vi "Main.vi"() -> ()   [LabVIEW 2009]
uses:
  <vilib>/Instr/_visa.llb/VISA Configure Serial Port (Instr).vi
panel:
  out "x-y":u32
  out "String":string
  in  "偵測數值":bool
  out "Cluster":T1={"試驗速度"=10, "加速時間"=10, "試驗次數"=5000, "輪胎直徑"=1000, "異常煞車時間"=50}
  in  "stop":bool
  in  "偵測開啟":bool
  in  "控制開啟":bool
  in  "Y10~Y17":bool[](array[boolean])=[FALSE, FALSE, FALSE, FALSE, FALSE, FALSE, FALSE, FALSE]
  in  "Y0~Y7":bool[](array[boolean])=[FALSE, FALSE, FALSE, FALSE, FALSE, FALSE, FALSE, FALSE]
  out "X10~X17":bool[](array[boolean])
  out "X0~X7":bool[](array[boolean])
  in  "COM Port":refnum<visa-resource-name>="COM6"
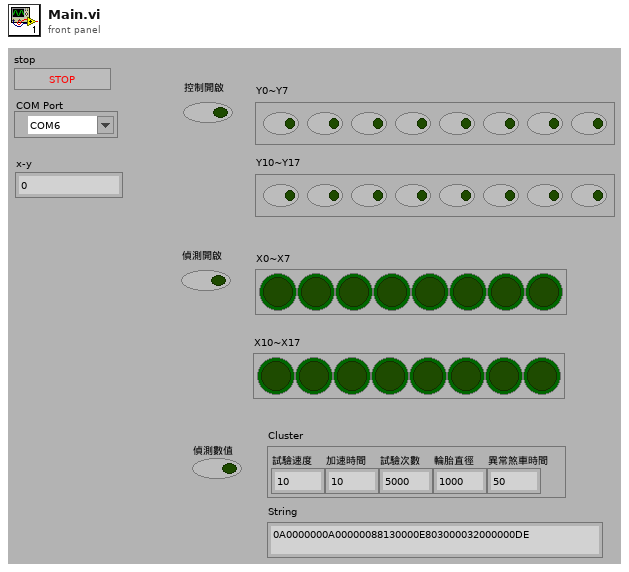
[diagram p1: front panel]
types:
  T1 = cluster{"試驗速度":u32, "加速時間":u32, "試驗次數":u32, "輪胎直徑":u32, "異常煞車時間":u32}
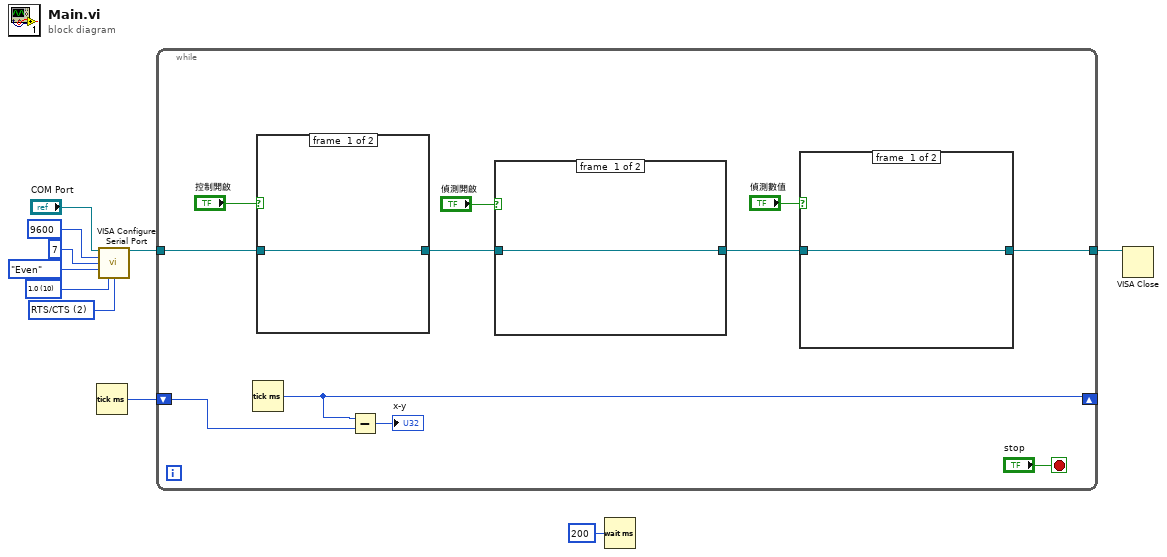
[diagram p0: block diagram]
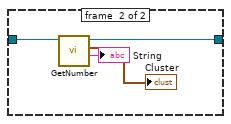
[diagram p2: hidden frame]
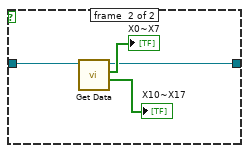
[diagram p3: hidden frame]
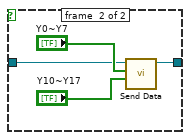
[diagram p4: hidden frame]
diagram:
  w6 = u16 2 items=["None", "XON/XOFF", "RTS/CTS", "XON/XOFF & RTS/CTS", "DTR/DSR", "XON/XOFF & DTR/DSR"] ("flow control (0:none)")
  w7 = u16 10 items=["1.0"=10, "1.5"=15, "2.0"=20] ("stop bits (10: 1 bit)")
  n1 = Tick Count (ms)() -> (millisecond timer value=w1:u32)
  n2 = call-poly "VISA Configure Serial Port"("VISA resource name"="COM Port", "baud rate (9600)"=u32 9600, "data bits (8)"=u16 7, "parity (0:none)"=enum16{"None", "Odd", "Even", "Mark", "Space"}."Even", "stop bits (10: 1 bit)"=w7, "flow control (0:none)"=w6) -> ("VISA resource name out"=w4:refnum<visa-resource-name>)  [unwired: 8 in, 1 out]
  n3 = while {
    tunnel: w4 -> [w19]
    tunnel: [w15] -> w3
    shift-right: [w13] -> _
    shift-left: w1 -> [w12]
    stop <- "stop" stop-if-true
    n4 = Tick Count (ms)() -> (millisecond timer value=w13:u32)
    n5 = case shown="True" "控制開啟" {
      tunnel: w19 -> [w32 w34]
      tunnel: [w32 w33] -> w17
      frame #0 {
      }
      frame #1 {
        n6 = call "Send Data.vi"("Array 2"="Y10~Y17", "Array"="Y0~Y7", "VISA Input"=w34) -> ("VISA Output"=w33:refnum<visa-resource-name>)  [unwired: 8 in]
      }
    }
    n7 = Subtract(x=w13, y=w12) -> (x-y=→"x-y":u32)
    n8 = case shown="True" "偵測開啟" {
      tunnel: w17 -> [w27 w29]
      tunnel: [w27 w28] -> w16
      frame #0 {
      }
      frame #1 {
        n9 = call "Get Data.vi"("VISA Input"=w29) -> ("X10~X17"=→"X10~X17":bool[], "X0~X7"=→"X0~X7":bool[], "VISA Output"=w28:refnum<visa-resource-name>)  [unwired: 7 in, 1 out]
      }
    }
    n10 = case shown="True" "偵測數值" {
      tunnel: w16 -> [w22 w25]
      tunnel: [w22 w24] -> w15
      frame #0 {
      }
      frame #1 {
        n11 = call "GetNumber.vi"("COM Port"=w25) -> ("String"=→"String":string, "Cluster"=→"Cluster":T1, "VISA Output"=w24:refnum<visa-resource-name>)  [unwired: 8 in]
      }
    }
  }
  n12 = Wait (ms)(milliseconds to wait=u32 200) -> ()  [unwired: 1 out]
  n13 = VISA Close(VISA resource name=w3) -> ()  [unwired: 1 in, 1 out]
